vi "Homework_3_Exact.vi"() -> ()   [LabVIEW 2011]
uses:
  <vilib>/imath/engines/lvmath/Plug In/_Char/NIMS_CH_character datatype.ctl
  <vilib>/imath/engines/lvmath2/RunTimeEngine/ErrorHandling/NIMS_Finalize Error.vi
  <vilib>/imath/engines/lvmath2/RunTimeEngine/Managers/WorkSpace/UID Generator.vi
  <vilib>/imath/engines/lvmath2/RunTimeEngine/VariableToken/NIMS_VariableToken_CondDefined.vi
  <instcachedir>/0/NIMS_VariableToken_CondDefined_D30D2F4D3CE04567BC79CC35D27951F7.lvgen/NIMS_VariableToken_CondDefined_D30D2F4D3CE04567BC79CC35D27951F7_000.vi
  <vilib>/imathl/engines/lvmath/Functions/Error Handling/Create Error.vi
  <vilib>/imath/engines/lvmath/Functions/Error Handling/MergeErrorsWrapper.vi
  <vilib>/imath/engines/lvmath2/RunTimeEngine/Managers/SymbolTable/Clear UID.vi
  <vilib>/imath/engines/lvmath2/RunTimeEngine/NodeEndStatement/NIMS_NodeEndStatement_Output.vi
  <instcachedir>/0/NIMS_NodeEndStatement_Output_53EC0D466D134D7ABD903AC30B43404B.lvgen/NIMS_NodeEndStatement_Output_53EC0D466D134D7ABD903AC30B43404B_005.vi
  <instcachedir>/0/NIMS_NodeEndStatement_Output_53EC0D466D134D7ABD903AC30B43404B.lvgen/NIMS_NodeEndStatement_Output_53EC0D466D134D7ABD903AC30B43404B_000.vi
  <vilib>/imath/engines/lvmath2/RunTimeEngine/BuiltInFunctions/atan2/NIMS_atan2.vi
  <instcachedir>/0/NIMS_atan2_A91AA4A7D42247EDBE8F76DB99AF04A4.lvgen/NIMS_atan2_A91AA4A7D42247EDBE8F76DB99AF04A4_000.vi
  <instcachedir>/0/NIMS_atan2_A91AA4A7D42247EDBE8F76DB99AF04A4.lvgen/NIMS_atan2_A91AA4A7D42247EDBE8F76DB99AF04A4_001.vi
  <vilib>/imath/engines/lvmath2/RunTimeEngine/BuiltInFunctions/asin/NIMS_asin(C).vi
  <instcachedir>/0/NIMS_asin(C)_6306C66EBAF1432D964D70ABF47AB540.lvgen/NIMS_asin(C)_6306C66EBAF1432D964D70ABF47AB540_001.vi
  <vilib>/imath/engines/lvmath2/RunTimeEngine/RangeToken/NIMS_Range_R2 - Integer.vi
  <instcachedir>/0/NIMS_Range_R2 - Integer_8B99B1FAA0BB43C693F13B8216F464EC.lvgen/NIMS_Range_R2 - Integer_8B99B1FAA0BB43C693F13B8216F464EC_000.vi
  <vilib>/imath/engines/lvmath2/RunTimeEngine/CommandStatement/MC_CommandStatement_break.vi
  <vilib>/imath/engines/lvmath2/RunTimeEngine/VariableToken/NIMS_VariableToken_CondDefinedDefinedByReplace.vi
  <instcachedir>/0/NIMS_VariableToken_CondDefinedDefinedByReplace_D162CFFC24174562A9FEA619A91E1A56.lvgen/NIMS_VariableToken_CondDefinedDefinedByReplace_D162CFFC24174562A9FEA619A91E1A56_000.vi
  <vilib>/imath/engines/lvmath2/RunTimeEngine/ReplaceToken/NIMS_Replace - Check Linear.vi
  <instcachedir>/0/NIMS_Replace - Check Linear_276AD648BD064726893CCF9ED6E2A728.lvgen/NIMS_Replace - Check Linear_276AD648BD064726893CCF9ED6E2A728_002.vi
  <vilib>/imath/engines/lvmath2/RunTimeEngine/VariableToken/Read/NIMS_Get Elements - RV(_) - Check.vi
  <instcachedir>/0/NIMS_Get Elements - RV(_) - Check_B511B9D8E05044FE80F9F088FE24B20C.lvgen/NIMS_Get Elements - RV(_) - Check_B511B9D8E05044FE80F9F088FE24B20C_000.vi
  <vilib>/imath/engines/lvmath2/RunTimeEngine/BuiltInFunctions/sin/NIMS_sin(C).vi
  <instcachedir>/0/NIMS_sin(C)_919C128BFD70440CAFCE8DBD597E0C76.lvgen/NIMS_sin(C)_919C128BFD70440CAFCE8DBD597E0C76_001.vi
  <vilib>/imath/engines/lvmath2/RunTimeEngine/ReplaceToken/NIMS_Replace - Size Check _(_)=S.vi
  <instcachedir>/0/NIMS_Replace - Size Check _(_)=S_9ABE7AF2D26C43EAA05192D5C1E6C624.lvgen/NIMS_Replace - Size Check _(_)=S_9ABE7AF2D26C43EAA05192D5C1E6C624_001.vi
  <vilib>/imath/engines/lvmath2/RunTimeEngine/ReplaceToken/NIMS_Replace - V(S)=S.vi
  <instcachedir>/0/NIMS_Replace - V(S)=S_16B13A4565AB46F59881314645612498.lvgen/NIMS_Replace - V(S)=S_16B13A4565AB46F59881314645612498_001.vi
  <vilib>/imath/engines/lvmath2/RunTimeEngine/ErrorHandling/NIMS_Create Error From Enums.vi
  <vilib>/imath/engines/lvmath2/RunTimeEngine/BuiltInFunctions/figure/NIMS_figure(I32).vi
  <vilib>/imath/engines/lvmath2/RunTimeEngine/BuiltInFunctions/plot/NIMS_plot(RM, RM, Str).vi
  <vilib>/imath/engines/lvmath/Plug In/_Char/NIMS_CH_Character RV to String.vi
  <vilib>/imath/engines/lvmath2/RunTimeEngine/BuiltInFunctions/legend/NIMS_legend(Arb).vi
  <vilib>/imath/engines/lvmath2/RunTimeEngine/BuiltInFunctions/ylabel/NIMS_ylabel.vi
  <vilib>/imath/engines/lvmath2/RunTimeEngine/BuiltInFunctions/xlabel/NIMS_xlabel.vi
  <vilib>/imath/engines/lvmath2/RunTimeEngine/Managers/SymbolTable/NIMS_WorkSpace.lvlib
panel:
  out "XY Graph":cluster{dbl[], dbl[]}[](graph)
  in  "Natural Frequency":dbl=25.0
  in  "Damping\nCoeffiencent":dbl=0.12
  in  "Frequency":dbl=38.0
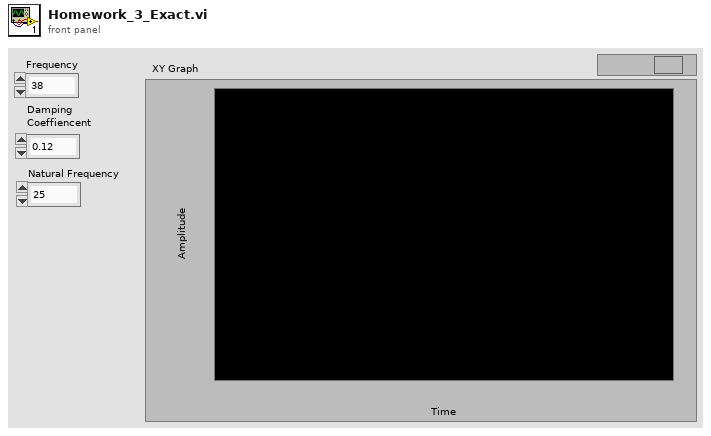
[diagram p1: front panel]
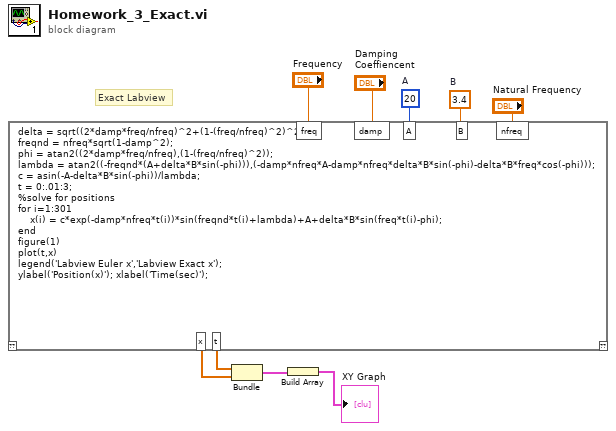
[diagram p0: block diagram]
diagram:
  w5 = 3.4  # B
  w6 = 20  # A
  # "Exact Labview"
  n1 = mathscript code="delta = sqrt((2*damp*freq/nfreq)^2+(1-(freq/nfreq)^2)^2);\nfreqnd = nfreq*sqrt(1-damp^2);\nphi = atan2((2*damp*freq/nfreq),(1-(freq/nfreq)^2));\nlambda = atan2((-freqnd*(A+delta*B*sin(-phi))),(-damp*nfreq*A-damp*nfreq*delta*B*sin(-phi)-delta*B*freq*cos(-phi)));\nc = asin(-A-delta*B*sin(-phi))/lambda;\nt = 0:.01:3;\n%solve for positions\nfor i=1:301\n    x(i) = c*exp(-damp*nfreq*t(i))*sin(freqnd*t(i)+lambda)+A+delta*B*sin(freq*t(i)-phi);\nend\nfigure(1)\nplot(t,x)\nlegend('Labview Euler x','Labview Exact x');\nylabel('Position(x)'); xlabel('Time(sec)');"("A"=w6, "B"=w5, "freq"="Frequency", "nfreq"="Natural Frequency", "damp"="Damping\nCoeffiencent") -> ("x"=w4:cdb[], "t"=w3:dbl[])  [unwired: 1 in, 1 out]
  n2 = Bundle("t"=w3, "x"=w4) -> (w2:cluster{"t":dbl[], "x":cdb[]})  [unwired: 1 in]
  n3 = Build Array(w2) -> (→"XY Graph":cluster{"t":dbl[], "x":cdb[]}[])
